vi "getEposInCurrentUnits.vi"(8 "error in (no error)":errorcluster, 10 "Axis Letter":string, 11 "Controller in":refnum<class "Controller.lvclass">) -> (0 "error out":errorcluster, 2 "EPOS In Current Units":dbl, 3 "Controller out":refnum<class "Controller.lvclass">)   [LabVIEW 2019, in "Controller.lvclass"]
uses:
  Controller.lvclass
  Axis/Axis.lvclass
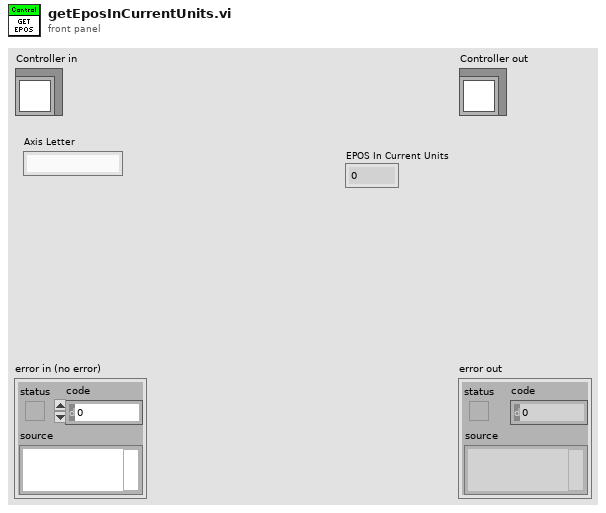
[diagram p1: front panel]
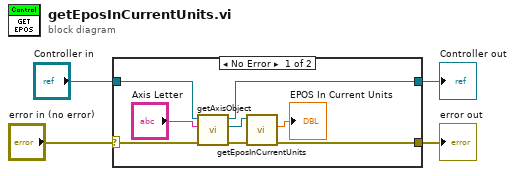
[diagram p0: block diagram]
diagram:
  n1 = case shown="No Error" "error in (no error)" {
    selector: "error in (no error)" -> [w8 w14]
    tunnel: [w6 w14] -> w3
    tunnel: [w9 w13] -> w1
    tunnel: "Controller in" -> [w11 w13]
    frame No Error {
      n2 = call-dynamic "getAxisObject.vi"("error in (no error)"=w8, "Axis Letter"="Axis Letter", "Controller in"=w11) -> ("error out"=w7:errorcluster, "Axis Object"=w12:refnum<class "Axis.lvclass">, "Controller out"=w9:refnum<class "Controller.lvclass">)  [unwired: 6 in]
      n3 = call-dynamic "getEposInCurrentUnits.vi"("error in (no error)"=w7, "Axis in"=w12) -> ("error out"=w6:errorcluster, "EPOS In Current Units"=→"EPOS In Current Units":dbl)  [unwired: 7 in, 1 out]
    }
    frame Error {
    }
  }
  "error out" <- w3
  "Controller out" <- w1
